vi "inclineCalibrate.vi"(8 "error in (no error)":errorcluster, 11 "VISA Refnum in":refnum<visa-resource-name>) -> (0 "error out":errorcluster, 2 "Elapsed Time (s)":dbl, 3 "Complete":bool=TRUE)   [LabVIEW 2018]
panel:
  in  "CycleCounter":i32
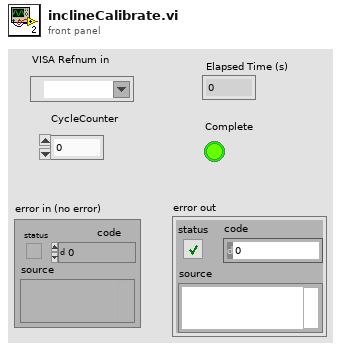
[diagram p1: front panel]
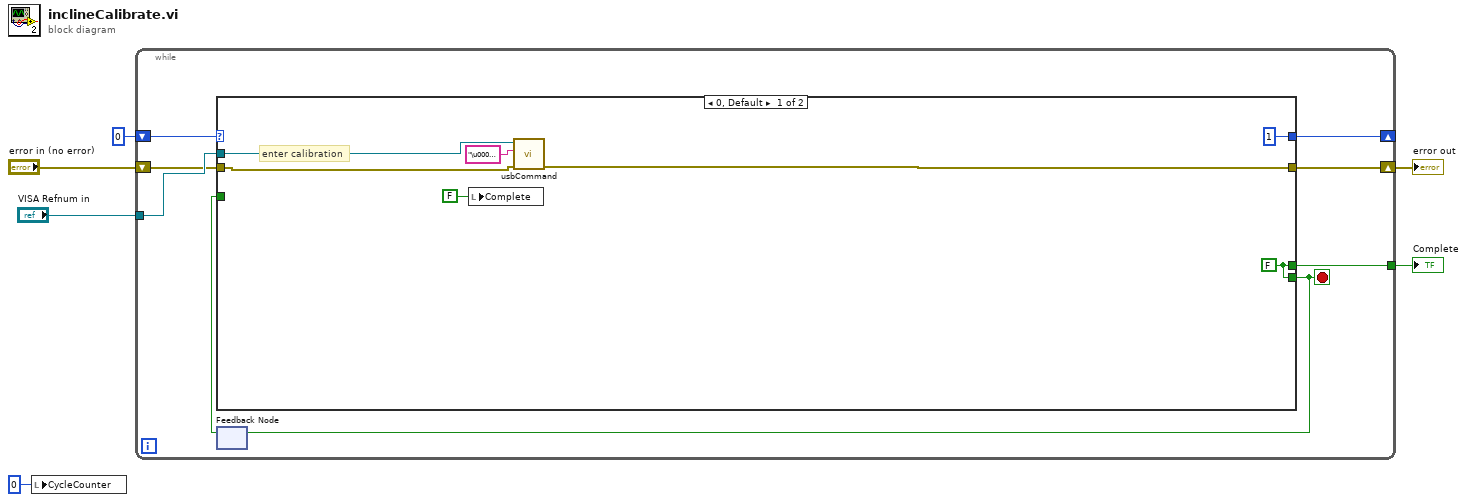
[diagram p0: block diagram]
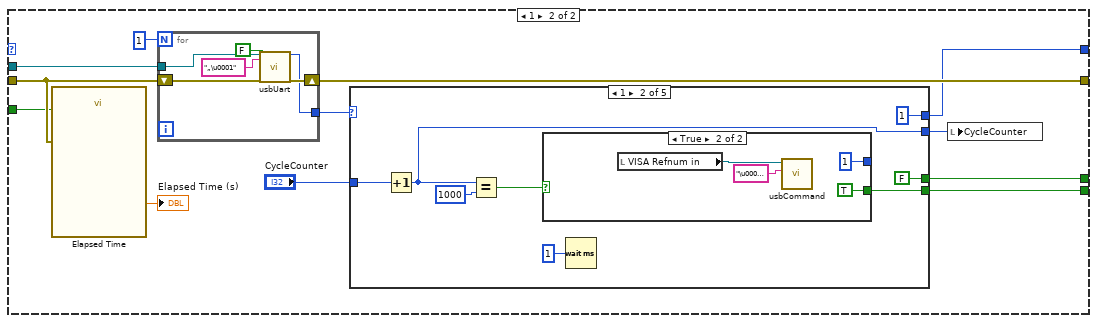
[diagram p2: hidden frame]
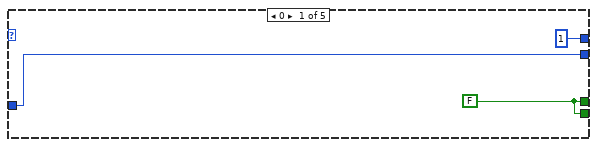
[diagram p3: hidden frame]
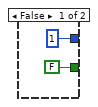
[diagram p4: hidden frame]
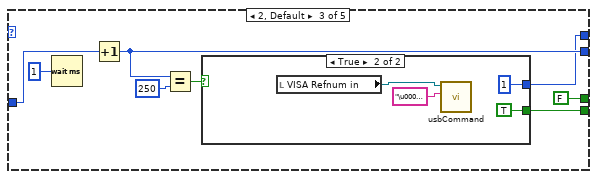
[diagram p5: hidden frame]
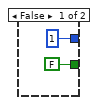
[diagram p6: hidden frame]
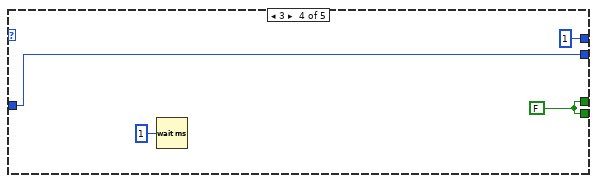
[diagram p7: hidden frame]
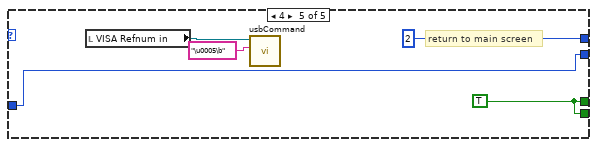
[diagram p8: hidden frame]
diagram:
  n1 = local write "CycleCounter"(0) -> ()
  n2 = while {
    tunnel: "VISA Refnum in" -> [w13]
    shift-right: [w12] -> _
    shift-left: 0 -> [w14]
    shift-right: [w10] -> w3
    shift-left: "error in (no error)" -> [w11]
    tunnel: [w9] -> w2
    stop <- w8 stop-if-true
    n3 = feedback #1() -> (w7:bool)  [unwired: 1 in]
    n4 = case shown="0, Default" w14 {
      tunnel: w13 -> [w20 w33]
      tunnel: [w16 w26] -> w8
      tunnel: [1 w31] -> w12
      tunnel: w11 -> [w18 w24]
      tunnel: [w17 w32] -> w10
      tunnel: [w16 w30] -> w9
      tunnel: w7 -> [_ w22]
      frame 0, Default {
        w16 = FALSE
        # "enter calibration"
        n5 = local write "Complete"(FALSE ("Complete")) -> ()
        n6 = call "usbCommand.vi"("error in (no error)"=w18, "write buffer"="\u0005\u0002", "VISA resource name in"=w20) -> ("error out"=w17:errorcluster)  [unwired: 7 in, 1 out]
      }
      frame 1 {
        n7 = call "Elapsed Time"("Reset"=w22, "error in (no error)"=w24) -> ("Elapsed Time (s)"=→"Elapsed Time (s)":dbl)  [unwired: 10 in, 7 out]
        n8 = for {
          N: 1 -> [_]
          tunnel: w33 -> [w38]
          tunnel: [w35] -> w28
          shift-right: [w36] -> w32
          shift-left: w24 -> [w37]
          n9 = call "usbUart.vi"("VISA resource name"=w38, "write buffer"="„\u0001", "sdFeature"=FALSE, "error in (no error)"=w37) -> ("number[0]"=w35:u32, "error out"=w36:errorcluster)  [unwired: 14 out]
        }
        n10 = case shown="1" w28 {
          tunnel: [1 1 w58 1 2] -> w31
          tunnel: [w40 FALSE FALSE w73 w75] -> w30
          tunnel: "CycleCounter" -> [w41 w49 w63 w74 w76]
          tunnel: [w41 w47 w61 w74 w76] -> w27
          tunnel: [w40 w43 w57 w73 w75] -> w26
          frame 0 {
            w40 = FALSE
          }
          frame 1 {
            n11 = Increment(x=w49) -> (x+1=w47:i32)
            n12 = Equal?(x=w47, y=1000) -> (x = y?=w45:bool)
            n13 = case shown="True" w45 {
              tunnel: [1 1] -> _
              tunnel: [FALSE TRUE] -> w43
              frame False {
              }
              frame True {
                n14 = local read "VISA Refnum in"() -> (w53:refnum<visa-resource-name>)
                n15 = call "usbCommand.vi"("write buffer"="\u0005\u0002", "VISA resource name in"=w53) -> ()  [unwired: 8 in, 2 out]
              }
            }
            n16 = Wait (ms)(milliseconds to wait=u32 1) -> ()  [unwired: 1 out]
          }
          frame 2, Default {
            n17 = Wait (ms)(milliseconds to wait=u32 1) -> ()  [unwired: 1 out]
            n18 = Increment(x=w63) -> (x+1=w61:i32)
            n19 = Equal?(x=w61, y=250) -> (x = y?=w59:bool)
            n20 = case shown="True" w59 {
              tunnel: [1 1] -> w58
              tunnel: [FALSE TRUE] -> w57
              frame False {
              }
              frame True {
                n21 = local read "VISA Refnum in"() -> (w67:refnum<visa-resource-name>)
                n22 = call "usbCommand.vi"("write buffer"="\u0005\u0002", "VISA resource name in"=w67) -> ()  [unwired: 8 in, 2 out]
              }
            }
          }
          frame 3 {
            w73 = FALSE
            n23 = Wait (ms)(milliseconds to wait=u32 1) -> ()  [unwired: 1 out]
          }
          frame 4 {
            w75 = TRUE
            # "return to main screen"
            n24 = local read "VISA Refnum in"() -> (w77:refnum<visa-resource-name>)
            n25 = call "usbCommand.vi"("write buffer"="\u0005\b", "VISA resource name in"=w77) -> ()  [unwired: 8 in, 2 out]
          }
        }
        n26 = local write "CycleCounter"(w27) -> ()
      }
    }
    n27 = feedback-in #1(w8) -> ()
  }
  "error out" <- w3
  "Complete" <- w2
